vi "scanRegionLogic.vi"() -> (0 "Error":bool)   [LabVIEW 2014]
uses:
  Controls/infoHandle.ctl
  <vilib>/rvi/Emulation/niFpgaGetClockAttributes.vi
  <vilib>/rvi/Emulation/niFpgaSctlEmulationGetInTimedLoop.vi
  <vilib>/rvi/Emulation/niFpgaEmulationReportErrorSimple.vi
  trackGlobVar.vi
  sequencerGlobVars.vi
  <vilib>/rvi/Emulation/niFpgaProcessEmulError.vi
  <vilib>/rvi/Emulation/niFpgaCriticalErrorInLSC.vi
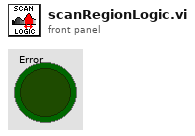
[diagram p1: front panel]
types:
  T1 = typedef "infoHandle.ctl" = enum16{"abortedScan", "stepComplete", "newScan", "newBunch"}
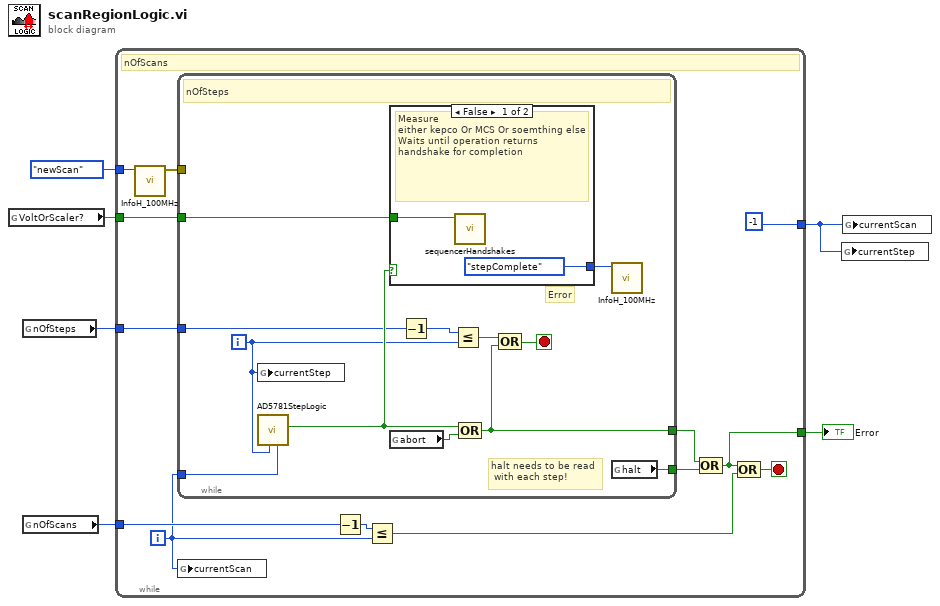
[diagram p0: block diagram]
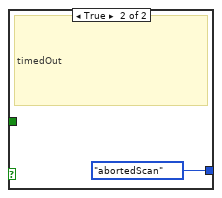
[diagram p2: hidden frame]
diagram:
  n1 = global read "trackGlobVar.vi" "VoltOrScaler?"() -> (w3:bool)
  n2 = global read "trackGlobVar.vi" "nOfSteps"() -> (w4:i32)
  n3 = global read "trackGlobVar.vi" "nOfScans"() -> (w5:i32)
  n4 = while {
    tunnel: [w12] -> w6
    tunnel: w5 -> [w16]
    tunnel: w4 -> [w15]
    tunnel: w3 -> [w14]
    tunnel: infoHandle."newScan" ("info") -> [w11]
    tunnel: [-1 ("currentScan")] -> w1
    i -> [w8]
    stop <- w18 stop-if-true
    # "nOfScans"
    n5 = call "InfoH_100MHz.vi"("info"=w11) -> ("Error"=w10:errorcluster)  [unwired: 10 in]
    n6 = while {
      tunnel: [w20] -> w13
      tunnel: w8 -> [w26]
      tunnel: w15 -> [w25]
      tunnel: w14 -> [w24]
      tunnel: w10 -> [_]
      tunnel: [w22] -> w9
      i -> [w21]
      stop <- w28 stop-if-true
      # "halt needs to be read\n with each step!"
      # "Error"
      # "nOfSteps"
      n7 = global write "sequencerGlobVars.vi" "currentStep"(w21) -> ()
      n8 = call "AD5781StepLogic.vi"("actTrack"=w26, "actStep"=w21) -> ("timedOut"=w30:bool)  [unwired: 9 in]
      n9 = case shown="False" w30 {
        tunnel: w24 -> [w33 _]
        tunnel: [infoHandle."stepComplete" ("info") infoHandle."abortedScan" ("info")] -> w23
        frame False {
          # "Measure\neither kepco Or MCS Or soemthing else\nWaits until operation returns handshake for completion"
          n10 = call "sequencerHandshakes.vi"("VoltOrScaler?"=w33) -> ()  [unwired: 11 in]
        }
        frame True {
          # "timedOut"
        }
      }
      n11 = global read "sequencerGlobVars.vi" "abort"() -> (w29:bool)
      n12 = Decrement(x=w25) -> (x-1=w31:i32)
      n13 = Less Or Equal?(x=w31, y=w21) -> (x <= y?=w27:bool)
      n14 = Compound Arithmetic op=OR(w30, w29) -> (w20:bool)
      n15 = Compound Arithmetic op=OR(w27, w20) -> (w28:bool)
      n16 = call "InfoH_100MHz.vi"("info"=w23) -> ()  [unwired: 10 in, 1 out]
      n17 = global read "sequencerGlobVars.vi" "halt"() -> (w22:bool)
    }
    n18 = global write "sequencerGlobVars.vi" "currentScan"(w8) -> ()
    n19 = Decrement(x=w16) -> (x-1=w17:i32)
    n20 = Less Or Equal?(x=w17, y=w8) -> (x <= y?=w19:bool)
    n21 = Compound Arithmetic op=OR(w13, w9) -> (w12:bool)
    n22 = Compound Arithmetic op=OR(w12, w19) -> (w18:bool)
  }
  "Error" <- w6
  n23 = global write "sequencerGlobVars.vi" "currentStep"(w1) -> ()
  n24 = global write "sequencerGlobVars.vi" "currentScan"(w1) -> ()
